vi "Control Check File.vi"(4 "RT Remote File Storage":bool, 5 "RT reference":refnum<vi>, 6 "RT Connected":bool, 7 "File Path":path) -> (0 "error out":errorcluster, 3 "File Out":path)   [LabVIEW 2023]
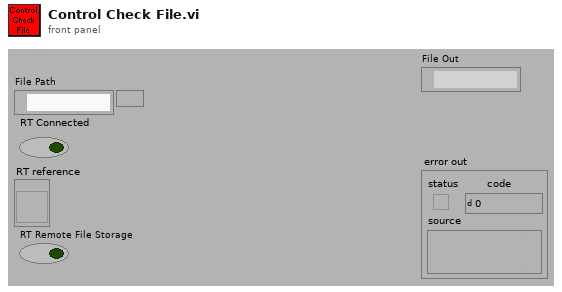
[diagram p1: front panel]
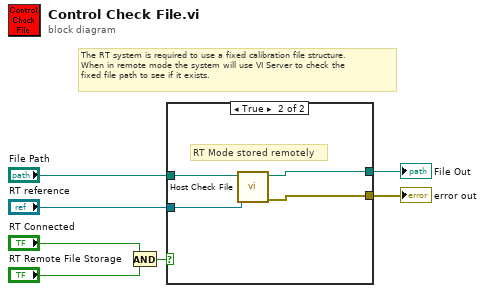
[diagram p0: block diagram]
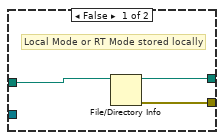
[diagram p2: hidden frame]
diagram:
  # "The RT system is required to use a fixed calibration file structure.\nWhen in remote mode the system will use VI Server to check the\nfixed file path to see if it exists."
  n1 = And(x="RT Connected", y="RT Remote File Storage") -> (x .and. y?=w2:bool)
  n2 = case shown="True" w2 {
    tunnel: [w10 w14] -> w7
    tunnel: "RT reference" -> [_ w12]
    tunnel: [w9 w13] -> w6
    tunnel: "File Path" -> [w8 w11]
    frame False {
      # "Local Mode or RT Mode stored locally"
      n3 = File/Directory Info(path=w8) -> (path out=w10:path, error out=w9:errorcluster)  [unwired: 1 in, 5 out]
    }
    frame True {
      # "RT Mode stored remotely"
      n4 = call "Host Check File.vi"("RT reference"=w12, "File Path"=w11) -> ("File error"=w13:errorcluster, "dup path"=w14:path)  [unwired: 7 in, 1 out]
    }
  }
  "File Out" <- w7
  "error out" <- w6
